vi "Leitura da Calibracao.vi"() -> (0 "min P 1":dbl, 1 "max P 1":dbl, 2 "min P 2":dbl, 3 "max P 2":dbl, 4 "min P 3":dbl, 5 "max P 3":dbl, 6 "min P 4":dbl, 7 "max P 4":dbl, 8 "min P 5":dbl, 9 "min P 8":dbl, 10 "max P 5":dbl, 11 "max P 8":dbl, 12 "min P 6":dbl, 13 "min P 9":dbl, 14 "max P 6":dbl, 15 "max P 9":dbl, 16 "min P 7":dbl, 17 "min P 10":dbl, 18 "max P 7":dbl, 19 "max P 10":dbl, 20 "min P 11":dbl, 21 "max P 11":dbl)   [LabVIEW 2019]
uses:
  <vilib>/Utility/file.llb/Read Delimited Spreadsheet (DBL).vi
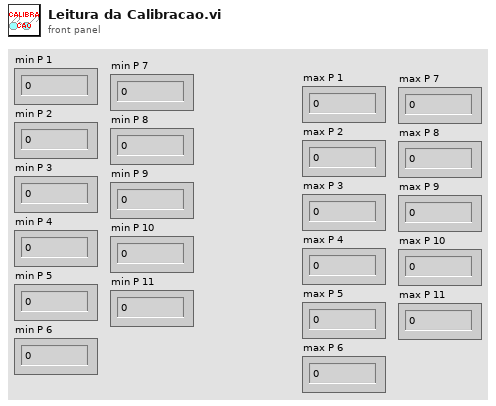
[diagram p1: front panel]
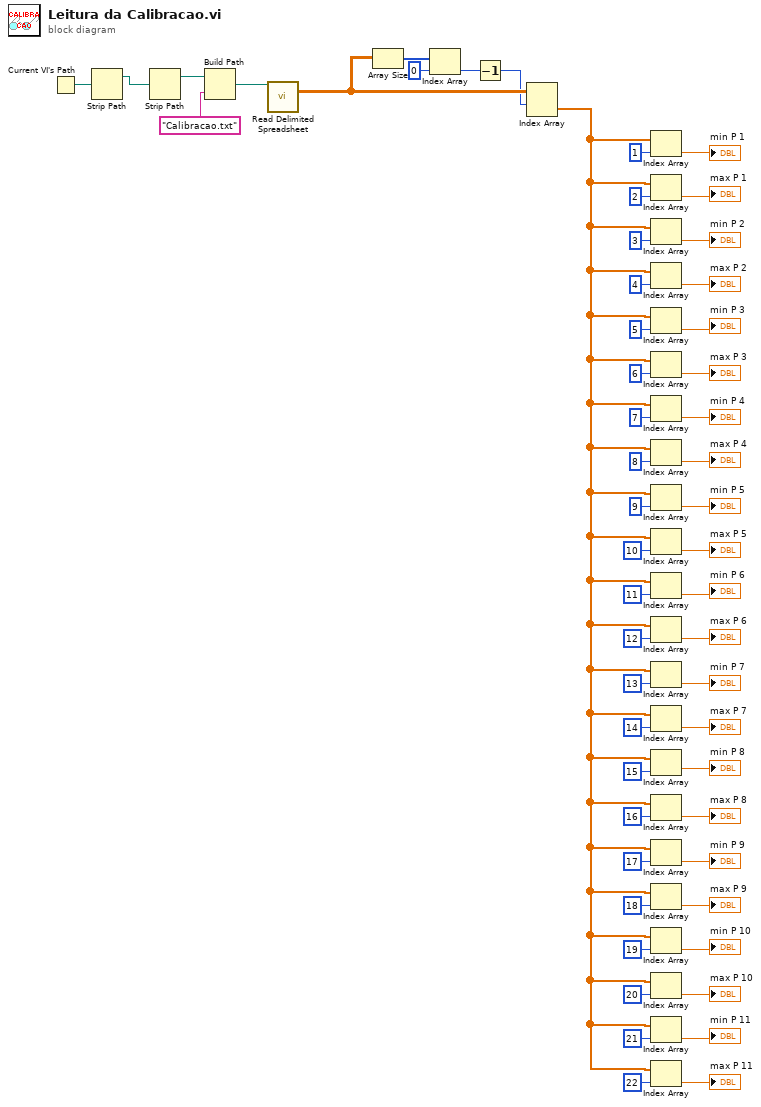
[diagram p0: block diagram]
diagram:
  n1 = Current VI's Path() -> (path=w54:path)
  n2 = Strip Path(path=w54) -> (stripped path=w52:path)  [unwired: 1 out]
  n3 = Strip Path(path=w52) -> (stripped path=w51:path)  [unwired: 1 out]
  n4 = Build Path(base path=w51, name or relative path="Calibracao.txt") -> (appended path=w55:path)
  n5 = call-poly <vilib>:"Read Delimited Spreadsheet.vi"("file path (dialog if empty)"=w55) -> ("all rows"=w48:dbl[][])  [unwired: 9 in, 5 out]
  n6 = Array Size(array=w48) -> (size(s)=w50:i32[])
  n7 = Index Array(array=w50, index=0) -> (element=w47:i32)
  n8 = Decrement(x=w47) -> (x-1=w46:i32)
  n9 = Index Array(array=w48, index (row)=w46) -> (element=w23:dbl[])  [unwired: 1 in]
  n10 = Index Array(array=w23, index=1) -> (element=→"min P 1":dbl)
  n11 = Index Array(array=w23, index=2) -> (element=→"max P 1":dbl)
  n12 = Index Array(array=w23, index=3) -> (element=→"min P 2":dbl)
  n13 = Index Array(array=w23, index=4) -> (element=→"max P 2":dbl)
  n14 = Index Array(array=w23, index=5) -> (element=→"min P 3":dbl)
  n15 = Index Array(array=w23, index=6) -> (element=→"max P 3":dbl)
  n16 = Index Array(array=w23, index=7) -> (element=→"min P 4":dbl)
  n17 = Index Array(array=w23, index=8) -> (element=→"max P 4":dbl)
  n18 = Index Array(array=w23, index=9) -> (element=→"min P 5":dbl)
  n19 = Index Array(array=w23, index=10) -> (element=→"max P 5":dbl)
  n20 = Index Array(array=w23, index=11) -> (element=→"min P 6":dbl)
  n21 = Index Array(array=w23, index=12) -> (element=→"max P 6":dbl)
  n22 = Index Array(array=w23, index=13) -> (element=→"min P 7":dbl)
  n23 = Index Array(array=w23, index=14) -> (element=→"max P 7":dbl)
  n24 = Index Array(array=w23, index=15) -> (element=→"min P 8":dbl)
  n25 = Index Array(array=w23, index=16) -> (element=→"max P 8":dbl)
  n26 = Index Array(array=w23, index=17) -> (element=→"min P 9":dbl)
  n27 = Index Array(array=w23, index=18) -> (element=→"max P 9":dbl)
  n28 = Index Array(array=w23, index=19) -> (element=→"min P 10":dbl)
  n29 = Index Array(array=w23, index=20) -> (element=→"max P 10":dbl)
  n30 = Index Array(array=w23, index=21) -> (element=→"min P 11":dbl)
  n31 = Index Array(array=w23, index=22) -> (element=→"max P 11":dbl)
